vi "Sample Power-DAQ-Stats.vi"() -> ()   [LabVIEW 2009]
uses:
  C:/Code/Apps/Utilities/PM2935/PMWinApp/PM_Installer/Master/Samples/1918 - 2936 Family/LabVIEW/LabVIEW 2009/PowerMeterCommands.dll
panel:
  in  "count":i32
  out "Device Key":string
  out "Std Dev Val":dbl
  out "Std Dev":string
  out "Range Val":dbl
  out "Range":string
  out "Mean Val":dbl
  out "Mean":string
  out "Min Val":dbl
  out "Min":string
  out "Max Val":dbl
  out "Max":string
  out "Data Acquisition":dbl[](array[numeric])
  out "Power Readings":string[](array[string])
  out "Status":string
  out "Power Value":dbl
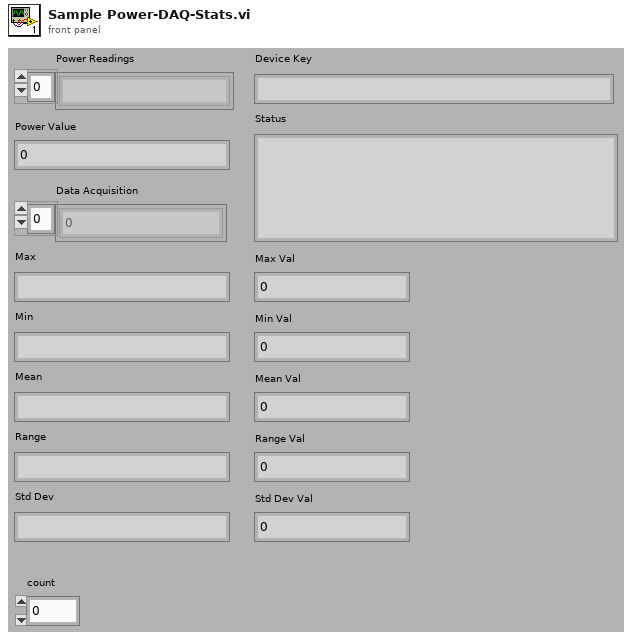
[diagram p1: front panel]
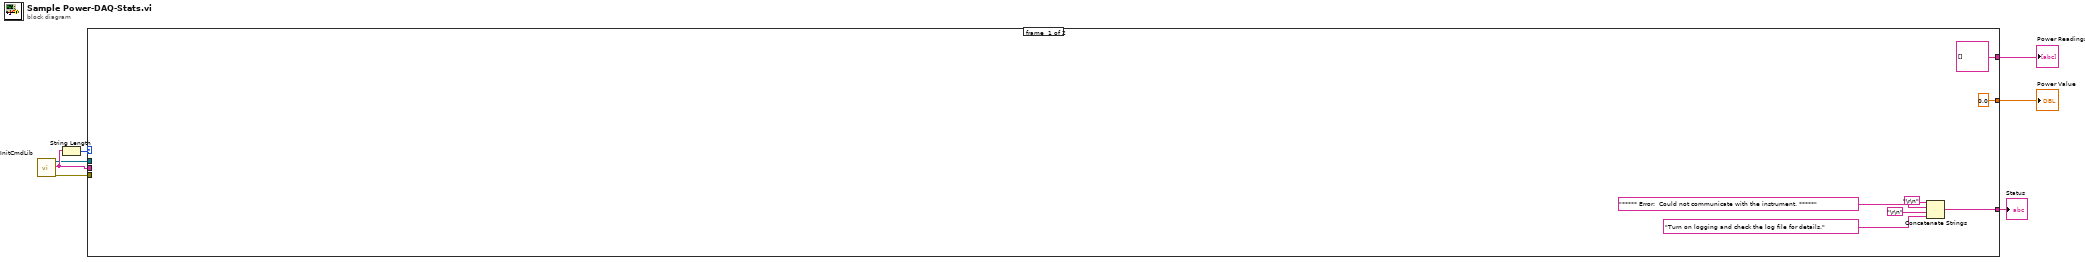
[diagram p0: block diagram]
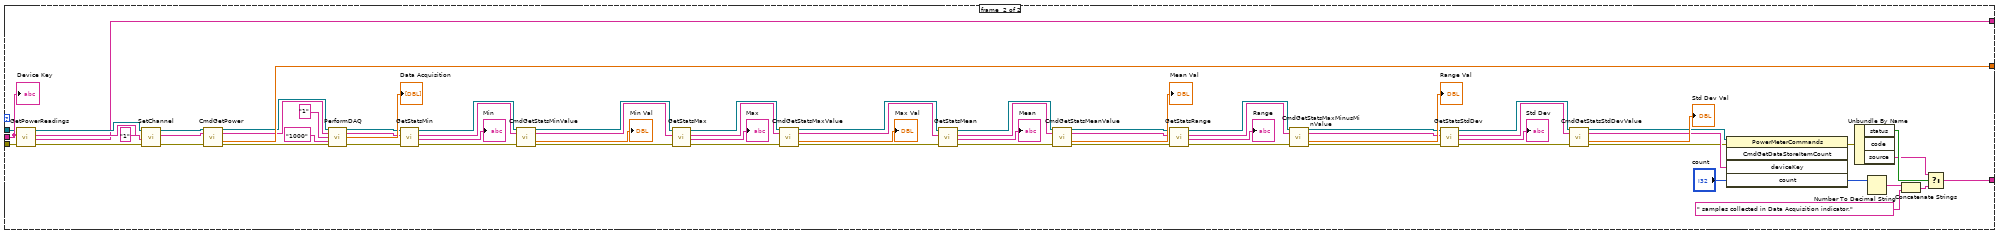
[diagram p2: hidden frame]
diagram:
  n1 = call "InitCmdLib.vi"() -> ("error out"=w2:errorcluster, "Device Key"=w3:string, "CmdLib"=w1:refnum<k24>)  [unwired: 9 in]
  n2 = String Length(string=w3) -> (length=w4:i32)
  n3 = case shown="1, Default" w4 {
    tunnel: [string[] [] ("Power Readings") w28] -> w7
    tunnel: [0.0 ("Power Value") w81] -> w6
    tunnel: [w8 w30] -> w5
    tunnel: w3 -> [_ w24]
    tunnel: w2 -> [_ w23]
    tunnel: w1 -> [_ w22]
    frame #0 {
      n4 = Concatenate Strings("\r\n", "***** Error:  Could not communicate with the instrument. *****", "\r\n", "Turn on logging and check the log file for details.") -> (w8:string)
    }
    frame #1 {
      n5 = call "GetPowerReadings.vi"("error in"=w23, "Device Key In"=w24, "PM Cmds In"=w22) -> ("error out"=w82:errorcluster, "Power Readings"=w28:string[], "Device Key Out"=w75:string, "PM Cmds Out"=w83:refnum<k24>)  [unwired: 1 in]
      n6 = call "SetChannel.vi"("error in"=w82, "Channel 1 or 2"="1" ("channel"), "Device Key In"=w75, "PM Cmds In"=w83) -> ("error out"=w72:errorcluster, "Device Key Out"=w71:string, "PM Cmds Out"=w73:refnum<k24>)  [unwired: 1 in]
      n7 = call "CmdGetPower.vi"("PM Cmds In"=w73, "Device Key In"=w71, "error in"=w72) -> ("PM Cmds Out"=w77:refnum<k24>, "Device Key Out"=w74:string, "Power Value"=w81:sgl, "error out"=w76:errorcluster)  [unwired: 8 in, 1 out]
      n8 = call "PerformDAQ.vi"("PM Cmds In"=w77, "Device Key In"=w74, "Interval"="1" ("interval"), "Sample Size"="1000" ("sampleSize"), "error in"=w76) -> ("PM Cmds Out"=w33:refnum<k24>, "Device Key Out"=w34:string, "Data Acquisition"=→"Data Acquisition":dbl[], "error out"=w27:errorcluster)  [unwired: 7 in]
      n9 = call "GetStatsMin.vi"("error in"=w27, "Device Key In"=w34, "PM Cmds In"=w33) -> ("error out"=w70:errorcluster, "Minimum"=→"Min":string, "Device Key Out"=w59:string, "PM Cmds Out"=w60:refnum<k24>)  [unwired: 5 in]
      n10 = call "CmdGetStatsMinValue.vi"("PM Cmds In"=w60, "Device Key In"=w59, "error in"=w70) -> ("PM Cmds Out"=w58:refnum<k24>, "Device Key Out"=w57:string, "Min Value"=→"Min Val":sgl, "error out"=w69:errorcluster)  [unwired: 8 in, 1 out]
      n11 = call "GetStatsMax.vi"("error in"=w69, "Device Key In"=w57, "PM Cmds In"=w58) -> ("error out"=w68:errorcluster, "Maximum"=→"Max":string, "Device Key Out"=w55:string, "PM Cmds Out"=w56:refnum<k24>)  [unwired: 5 in]
      n12 = call "CmdGetStatsMaxValue.vi"("PM Cmds In"=w56, "Device Key In"=w55, "error in"=w68) -> ("PM Cmds Out"=w54:refnum<k24>, "Device Key Out"=w53:string, "Max Value"=→"Max Val":sgl, "error out"=w67:errorcluster)  [unwired: 8 in, 1 out]
      n13 = call "GetStatsMean.vi"("error in"=w67, "Device Key In"=w53, "PM Cmds In"=w54) -> ("error out"=w66:errorcluster, "Mean"=→"Mean":string, "Device Key Out"=w51:string, "PM Cmds Out"=w52:refnum<k24>)  [unwired: 5 in]
      n14 = call "CmdGetStatsMeanValue.vi"("PM Cmds In"=w52, "Device Key In"=w51, "error in"=w66) -> ("PM Cmds Out"=w35:refnum<k24>, "Device Key Out"=w36:string, "Mean Value"=→"Mean Val":sgl, "error out"=w37:errorcluster)  [unwired: 8 in, 1 out]
      n15 = call "GetStatsRange.vi"("error in"=w37, "Device Key In"=w36, "PM Cmds In"=w35) -> ("error out"=w38:errorcluster, "Range"=→"Range":string, "Device Key Out"=w39:string, "PM Cmds Out"=w40:refnum<k24>)  [unwired: 5 in]
      n16 = call "CmdGetStatsMaxMinusMinValue.vi"("PM Cmds In"=w40, "Device Key In"=w39, "error in"=w38) -> ("PM Cmds Out"=w41:refnum<k24>, "Device Key Out"=w42:string, "Range Value"=→"Range Val":sgl, "error out"=w43:errorcluster)  [unwired: 8 in, 1 out]
      n17 = call "GetStatsStdDev.vi"("error in"=w43, "Device Key In"=w42, "PM Cmds In"=w41) -> ("error out"=w44:errorcluster, "Standard Deviation"=→"Std Dev":string, "Device Key Out"=w45:string, "PM Cmds Out"=w46:refnum<k24>)  [unwired: 5 in]
      n18 = call "CmdGetStatsStdDevValue.vi"("PM Cmds In"=w46, "Device Key In"=w45, "error in"=w44) -> ("PM Cmds Out"=w20:refnum<k24>, "Device Key Out"=w21:string, "Std Dev Value"=→"Std Dev Val":sgl, "error out"=w19:errorcluster)  [unwired: 8 in, 1 out]
      n19 = invoke class="PowerMeterCommands" method="CmdGetDataStoreItemCount"(reference=w20, error in=w19, "deviceKey"=w21, "count"="count") -> (error out=w15:errorcluster, "count"=w17:i32)  [unwired: 1 in, 3 out]
      n20 = Unbundle By Name(w15) -> ("status"=w31:bool, "source"=w29:string)  [unwired: 1 out]
      n21 = Number To Decimal String(number=w17) -> (decimal integer string=w16:string)  [unwired: 1 in]
      n22 = Concatenate Strings(w16, " samples collected in Data Acquisition indicator." ("string")) -> (w25:string)
      n23 = Select(t=w29, s=w31, f=w25) -> (s? t:f=w30:string)
      "Device Key" <- w24
    }
  }
  "Power Value" <- w6
  "Status" <- w5
  "Power Readings" <- w7
